vi "Init SLM Param v2.vi"() -> (1 "SLM Param Out":T1={"Error"={"status"=FALSE, "code"=0, "source"=""}, "References"={"Main VI"=refnum, "SLM VI"=refnum}, "Directories"={"Root Directory"=path "C:/Documents and Settings/tg273/My Documents/LabView VIs/Yale SLM/Yale v2/Mode Matrices", "Output Directory"=path "C:/Documents and Settings/tg273/My Documents/LabView VIs/Yale SLM/Yale v2/Mode Matrices"}, "Holo size"=504, "X pos"=-3, "Y pos"=-40, "Mode Coeffs"=[[2.0, 0.0], [3.0, 18.0], [4.0, 0.0], [11.0, 0.0], [22.0, 0.0], [37.0, 0.0], [5.0, 0.0], [6.0, 0.0], [7.0, 0.0], [8.0, 0.0], [9.0, 0.0], [10.0, 0.0]], "Wrap Value"=197, "Lambda (nm)"=750.0, "NA"=1.4, "Base Name"="", "Win Num"=2, "SLM SN"="0600535", "Holo Image Name"="0600535", "Matrix Name"="Unit Matrix.csv", "Mode Matrix"=array36x36[1296 elements], "Flatness"=array600x792[475200 elements], "STED Phase"=array504x504[254016 elements], "Ab Corr"=array504x504[254016 elements], "Holo Image"="remote image 000000000731AF64", "Holo Position"={-3.0, -40.0, 3840.0, 504.0}, "Apply Flatness\ncorr.?"=TRUE, "Max Wavelength (nm)"=750.0, "Min Wavelength (nm)"=750.0, "Vortex Rotation"=-3, "Top Hat Radius"=1.4, "SLM ID Num"="0600535", "Max Zernike Modes"=-3, "Screen Width"=2, "Ab Corr VI"={"AC VI Ref"=refnum, "# Modes"=2, "Mode Array"=[[4.0, 0.0, 0.0, 1.0, 0.0], [11.0, 0.75, 0.0, 1.0, 0.0], [22.0, 0.1, 0.0, 1.0, 0.0], [37.0, 0.0, 0.0, 1.0, 0.0], [7.0, 0.15, 0.0, 1.0, 0.0], [8.0, 0.1, 0.0, 1.0, 0.0], [5.0, 0.05, 0.0, 1.0, 0.0], [6.0, 0.0, 0.0, 1.0, 0.0], [9.0, 0.0, 0.0, 1.0, 0.0], [10.0, 0.0, 0.0, 1.0, 0.0], [2.0, 0.0, 0.0, 1.0, 0.0], [3.0, -18.3, 0.0, 1.0, 0.0]], "Apply Corr?"=TRUE, "Step Size"=0.3, "# Steps  "=11, "Resolution"=0.2, "FOV (um)"=12.0, "Metric Images"=[], "Metric Values"=[], "S"=[120.26, 128.5, 131.1, 136.15, 138.3, 148.05, 149.99, 150.02, 147.88, 152.65, 152.69, 150.56, 144.92, 143.08, 146.19, 140.15, 134.69, 125.47, 117.35, 108.32], "I"=[], "M"=[], "Coeff Steps"=[120.26, 128.5, 131.1, 136.15, 138.3, 148.05, 149.99, 150.02, 147.88, 152.65, 152.69, 150.56, 144.92, 143.08, 146.19, 140.15, 134.69, 125.47, 117.35, 108.32], "Mode Loop"={"Mode"=0, "Metric"=0, "Loop Index"=0}}} {"Vortex Rotation" format="%#_3g"; "Min Wavelength (nm)" format="%#_3g"; "Max Wavelength (nm)" format="%#_3g"; "Mode Matrix" format="%0.3f"; "Wrap Value" format="%#_3g"})   [LabVIEW 2014]
uses:
  TypeDefs/SLM Parameters.ctl
  <vilib>/vision/Image Controls.llb/IMAQ Image.ctl
types:
  T1 = typedef "SLM Parameters.ctl" = cluster{"Error":errorcluster, "References":cluster{"Main VI":refnum<vi>, "SLM VI":refnum<vi>}, "Directories":cluster{"Root Directory":path, "Output Directory":path}, "Holo size":u16, "X pos":i16, "Y pos":i16, "Mode Coeffs":dbl[][], "Wrap Value":i32, "Lambda (nm)":dbl, "NA":dbl, "Base Name":string, "Win Num":i32, "SLM SN":string, "Holo Image Name":string, "Matrix Name":string, "Mode Matrix":dbl[][], "Flatness":u8[][], "STED Phase":dbl[][], "Ab Corr":dbl[][], "Holo Image":T2, "Holo Position":cluster{dbl, dbl, dbl, dbl}, "Apply Flatness\ncorr.?":bool, "Max Wavelength (nm)":dbl, "Min Wavelength (nm)":dbl, "Vortex Rotation":i16, "Top Hat Radius":dbl, "SLM ID Num":string, "Max Zernike Modes":i16, "Screen Width":i32, "Ab Corr VI":cluster{"AC VI Ref":refnum<vi>, "# Modes":i32, "Mode Array":dbl[][], "Apply Corr?":bool, "Step Size":dbl, "# Steps  ":u16, "Resolution":dbl, "FOV (um)":dbl, "Metric Images":dbl[][][][], "Metric Values":dbl[][], "S":dbl[], "I":dbl[], "M":dbl[], "Coeff Steps":dbl[], "Mode Loop":cluster{"Mode":i8, "Metric":i8, "Loop Index":i8}}}
  T2 = typedef "IMAQ Image.ctl" = refnum<image>
  T3 = cluster{"X pos":i16, "Y pos":i16, i32, "Holo size":u16}
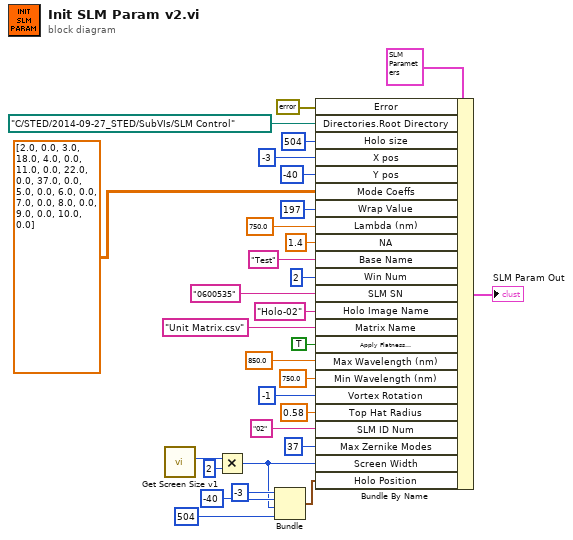
[diagram p0: block diagram]
diagram:
  n1 = call "Get Screen Size v1.vi"() -> ("Width"=w7:i32)  [unwired: 9 in, 2 out]
  n2 = Multiply(x=w7, y=2) -> (x*y=w2:i32)
  n3 = Bundle("X pos"=i16 -3, "Y pos"=i16 -40, w2, "Holo size"=u16 504) -> (w1:T3)  [unwired: 1 in]
  n4 = Bundle By Name(cluster=T1 {"Error"={"status"=FALSE, "code"=0, "source"=""}, "References"={"Main VI"=refnum, "SLM VI"=refnum}, "Directories"={"Root Directory"=path "", "Output Directory"=path ""}, "Holo size"=0, "X pos"=0, "Y pos"=0, "Mode Coeffs"=[], "Wrap Value"=0, "Lambda (nm)"=0.0, "NA"=0.0, "Base Name"="", "Win Num"=0, "SLM SN"="", "Holo Image Name"="", "Matrix Name"="", "Mode Matrix"=[], "Flatness"=[], "STED Phase"=[], "Ab Corr"=[], "Holo Image"=refnum, "Holo Position"={0.0, 0.0, 0.0, 0.0}, "Apply Flatness\ncorr.?"=FALSE, "Max Wavelength (nm)"=0.0, "Min Wavelength (nm)"=0.0, "Vortex Rotation"=0, "Top Hat Radius"=0.0, "SLM ID Num"="", "Max Zernike Modes"=0, "Screen Width"=0, "Ab Corr VI"={"AC VI Ref"=refnum, "# Modes"=0, "Mode Array"=[], "Apply Corr?"=FALSE, "Step Size"=0.0, "# Steps  "=0, "Resolution"=0.0, "FOV (um)"=0.0, "Metric Images"=[], "Metric Values"=[], "S"=[], "I"=[], "M"=[], "Coeff Steps"=[], "Mode Loop"={"Mode"=0, "Metric"=0, "Loop Index"=0}}} ("SLM Parameters"), "Error"=errorcluster {"status"=FALSE, "code"=0, "source"=""} ("error constant"), "Directories.Root Directory"=path "C:/STED/2014-09-27_STED/SubVIs/SLM Control" ("Mode Matrix Directory"), "Holo size"=u16 504, "X pos"=i16 -3, "Y pos"=i16 -40, "Mode Coeffs"=dbl[][] [[2.0, 0.0], [3.0, 18.0], [4.0, 0.0], [11.0, 0.0], [22.0, 0.0], [37.0, 0.0], [5.0, 0.0], [6.0, 0.0], [7.0, 0.0], [8.0, 0.0], [9.0, 0.0], [10.0, 0.0]], "Wrap Value"=u16 197 ("Holo size"), "Lambda (nm)"=750.0 ("Min Wavelength (nm)"), "NA"=1.4 ("lambda"), "Base Name"="Test", "Win Num"=i16 2 ("X pos"), "SLM SN"="0600535", "Holo Image Name"="Holo-02" ("Image Name"), "Matrix Name"="Unit Matrix.csv", "Apply Flatness\ncorr.?"=TRUE ("Apply Flatness\ncorr.?"), "Max Wavelength (nm)"=850.0, "Min Wavelength (nm)"=750.0 ("lambda"), "Vortex Rotation"=i16 -1, "Top Hat Radius"=0.58 ("lambda"), "SLM ID Num"="02" ("Image Name"), "Max Zernike Modes"=i16 37 ("Vortex Rotation"), "Screen Width"=w2, "Holo Position"=w1) -> (→"SLM Param Out":T1)
